vi "Speed Calculator.vi"(1 "Speed step":dbl=0.1, 2 "Previous Speed":dbl) -> (0 "New Speed":dbl)   [LabVIEW 2017]
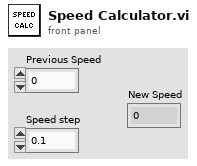
[diagram p1: front panel]
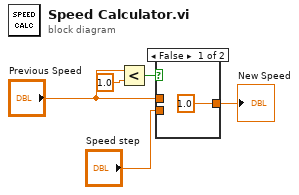
[diagram p0: block diagram]
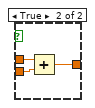
[diagram p2: hidden frame]
diagram:
  n1 = Less?(x="Previous Speed", y=1.0) -> (x < y?=w4:bool)
  n2 = case shown="False" w4 {
    tunnel: "Speed step" -> [_ w8]
    tunnel: "Previous Speed" -> [_ w9]
    tunnel: [1.0 w7] -> w1
    frame False {
    }
    frame True {
      n3 = Add(x=w9, y=w8) -> (x+y=w7:dbl)
    }
  }
  "New Speed" <- w1
